vi "Main.vi"(11 "Error in":errorcluster) -> (15 "Error out":errorcluster)   [LabVIEW 2020, in "PSRR Monitor.lvlib"]
uses:
  PSRR Monitor.lvlib
  Typedefs/Queue operations.ctl
  Typedefs/Data Cluster.ctl
  Typedefs/Variant cluster.ctl
  Typedefs/User LV2 operations.ctl
  Typedefs/User LV2 data.ctl
  <vilib>/Utility/config.llb/Read Key (I32).vi
  <vilib>/Utility/config.llb/Read Key (Boolean).vi
  SubVI/Error log.vi
  <vilib>/Utility/config.llb/Write Key (I32).vi
  <vilib>/Utility/config.llb/Write Key (Boolean).vi
  <vilib>/Utility/config.llb/NI_LVConfig.lvlib
panel:
  out "Obtained PSRR":i32(graph)
  in  "Error Log":bool
  in  "Exit":bool
  out "Description":string
  out "Time":string
  out "Type":string
  out "Error Code":i32
  out "Last Read PSRR (dB)":i32
  in  "Wait Time(sec)":i32 min=2 step=1
  out "Error?":bool
  # "PSRR MONITOR"
  # "Power Supply Rejection Ratio"
  # "Last Error Details"
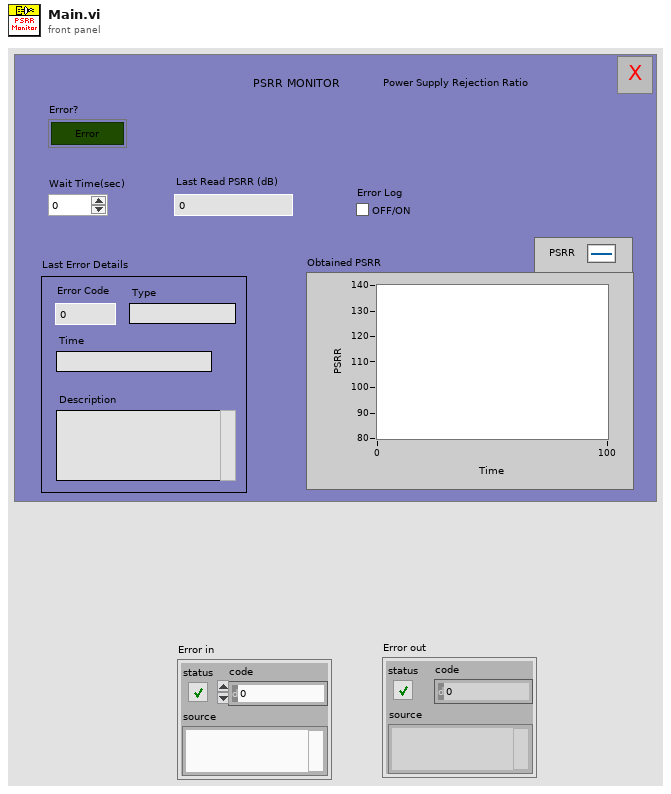
[diagram p1: front panel]
types:
  T1 = typedef "PSRR Monitor.lvlib/User LV2 operations.ctl" = enum16{"Destroy", "Get ref", "Generate", "Create"}
  T2 = typedef "PSRR Monitor.lvlib/Variant cluster.ctl" = cluster{"State":string, "Data":variant}
  T3 = typedef "PSRR Monitor.lvlib/Queue operations.ctl" = enum16{"Create", "Enqueue", "Enstack", "Dequeue", "Flush", "Release "}
  T4 = typedef "PSRR Monitor.lvlib/Data Cluster.ctl" = cluster{"Error?":bool, "Exit":bool, "Error log":bool, "Type":string, "Time":string, "Description":string, "Wait Time":i32, "Last Read PSRR":i32, "Error code":i32, "Obtained PSRR":i32, "Start/Stop Timer":bool, "Start time":dbl, "Path":path, "Passive count":dbl, "Other error count":dbl}
  T5 = typedef "PSRR Monitor.lvlib/User LV2 data.ctl" = cluster{"Exit":bool}
  T6 = typedef "NI_LVConfig.lvlib/Config Data RefNum.ctl" = refnum<k1>
  T7 = enum32{"Bad", "Idle", "Run top level", "Running"}
  T8 = typedef "PSRR Monitor.lvlib/Error Details.ctl" = cluster{"Error Code":i32, "Error Type":string, "Time":string, "Description":string, "PSRR":i32}
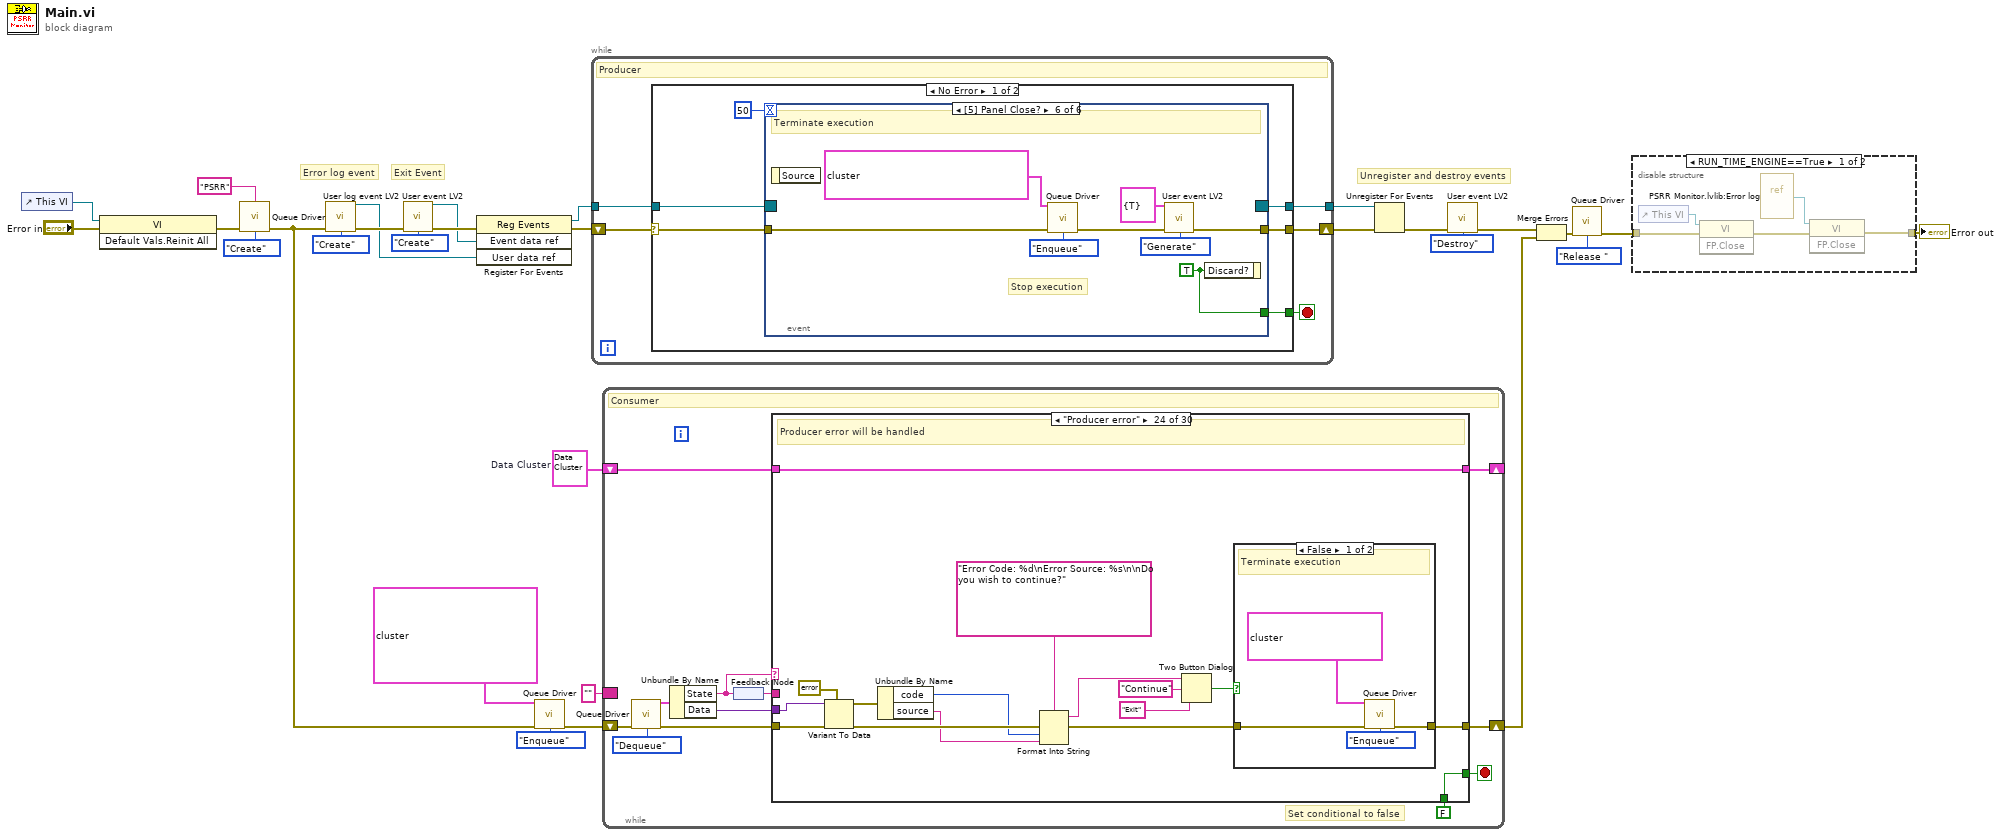
[diagram p0: block diagram]
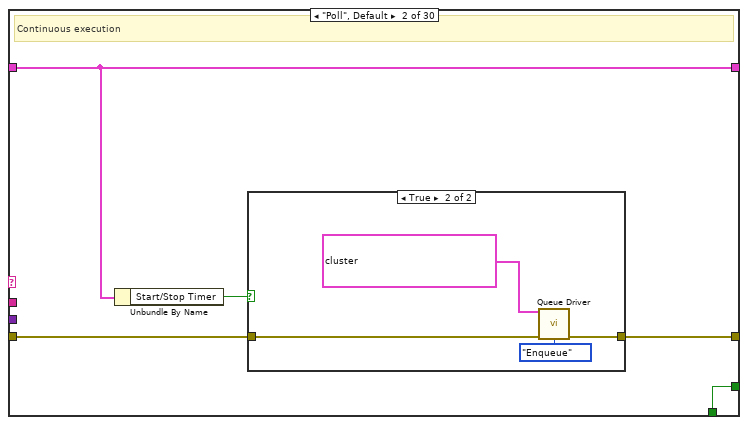
[diagram p4: hidden frame]
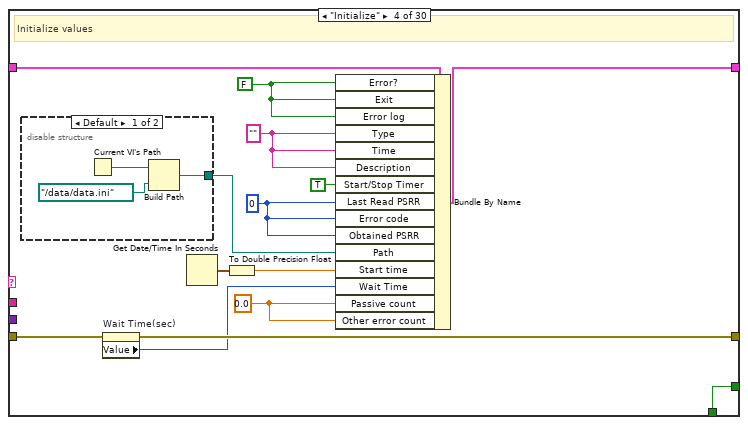
[diagram p7: hidden frame]
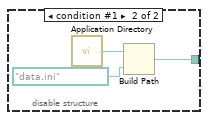
[diagram p8: hidden frame]
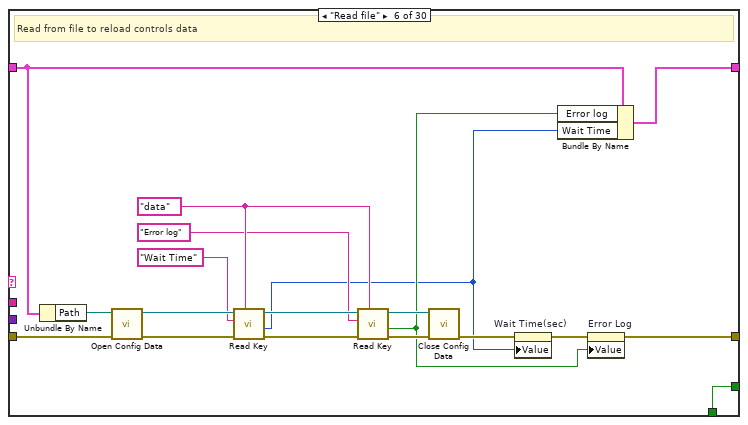
[diagram p10: hidden frame]
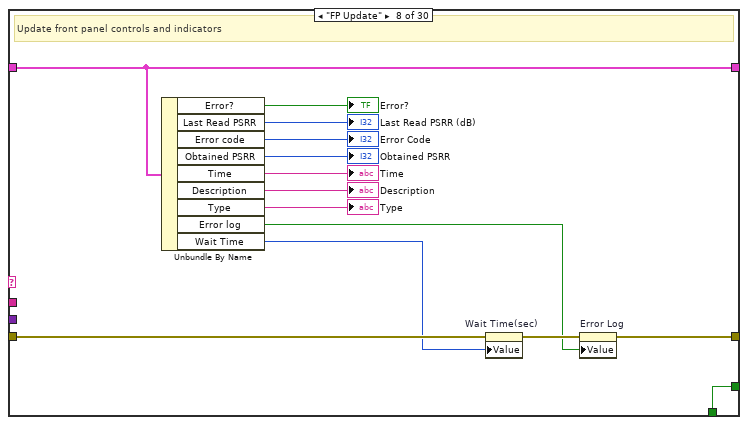
[diagram p12: hidden frame]
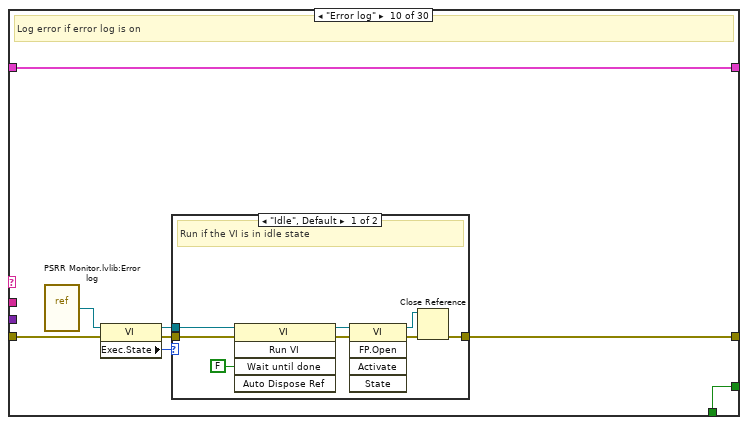
[diagram p14: hidden frame]
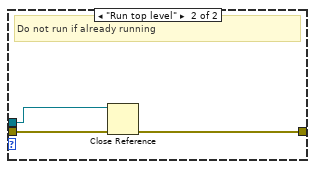
[diagram p15: hidden frame]
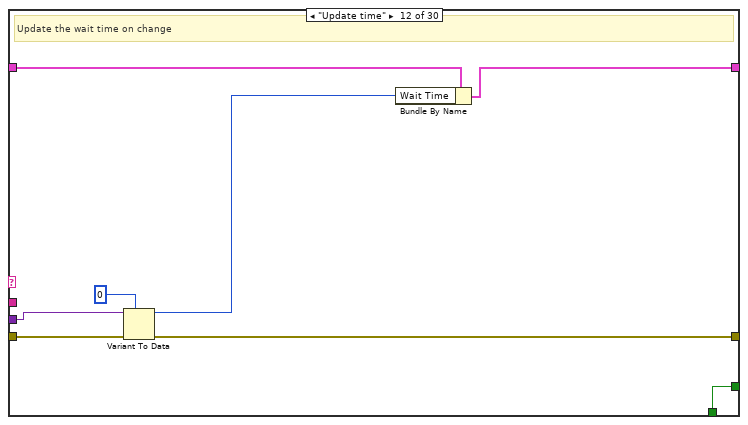
[diagram p17: hidden frame]
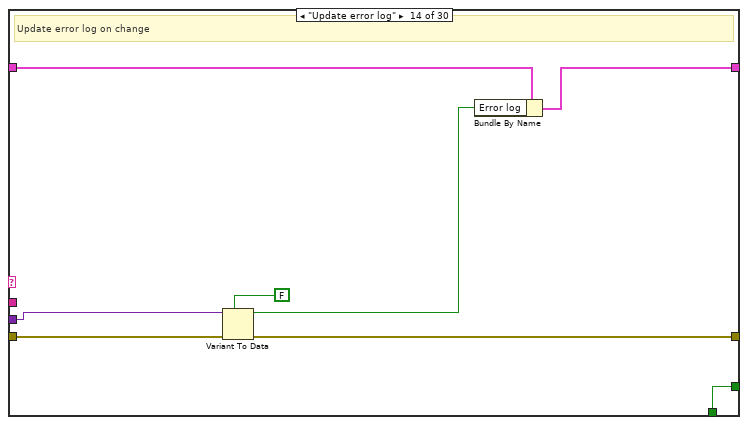
[diagram p19: hidden frame]
diagram:
  w24 = T4 {"Error?"=FALSE, "Exit"=FALSE, "Error log"=FALSE, "Type"="", "Time"="", "Description"="", "Wait Time"=0, "Last Read PSRR"=0, "Error code"=0, "Obtained PSRR"=0, "Start/Stop Timer"=FALSE, "Start time"=0.0, "Path"=path "", "Passive count"=0.0, "Other error count"=0.0}  # Data Cluster
  # "Unregister and destroy events"
  # "Exit Event"
  # "Error log event"
  n1 = control-ref of="This VI"() -> (w17:refnum<vi>)
  n2 = invoke class="VI" method="Default Vals.Reinit All"(reference=w17, error in="Error in") -> (error out=w15:errorcluster)  [unwired: 1 in, 2 out]
  n3 = call "Queue Driver.vi"("Name"="PSRR", "Error in"=w15, "Queue Operations"=Queue_operations."Create") -> ("Error out"=w3:errorcluster)  [unwired: 11 in, 1 out]
  n4 = call "User log event LV2.vi"("Error in"=w3, "Operation"=User_LV2_operations."Create") -> ("User data ref"=w1:refnum<user-event>, "Error out"=w2:errorcluster)  [unwired: 12 in]
  n5 = call "User event LV2.vi"("Error in"=w2, "Operation"=User_LV2_operations."Create") -> ("Event data ref"=w11:refnum<user-event>, "Error out"=w13:errorcluster)  [unwired: 12 in]
  n6 = register-events(error in=w13, w11, w1) -> (reference out=w10:refnum<event-registration>, error out=w12:errorcluster)  [unwired: 1 in]
  n7 = call "Queue Driver.vi"("State and data"=T2[] [{"State"="Initialize", "Data"=variant}, {"State"="Read file", "Data"=variant}, {"State"="FP Update", "Data"=variant}, {"State"="Error log", "Data"=variant}], "Error in"=w3, "Queue Operations"=Queue_operations."Enqueue") -> ("Error out"=w26:errorcluster)  [unwired: 11 in, 1 out]
  n8 = while {
    shift-right: [w33] -> w9
    shift-left: w12 -> [w34]
    tunnel: w10 -> [w31]
    tunnel: [w30] -> w8
    stop <- w32 stop-if-true
    # "Producer"
    n9 = case shown="No Error" w34 {
      selector: w34 -> [w38 w81]
      tunnel: [w39 w87] -> w33
      tunnel: [w37 FALSE ("Discard?")] -> w32
      tunnel: w31 -> [w36 w79]
      tunnel: [w35 w79] -> w30
      frame No Error {
        n10 = event shown="[5] Panel Close?" {
          selector: w36 -> [w41 _ _ _ _ _]
          dyn-events: [w41 _ _ _ _ _] -> w35
          timeout: 50 -> [_ _ _ _ _ _]
          tunnel: [w43 w50 w55 w65 w66 w71] -> w39
          tunnel: w38 -> [w43 w51 w56 w65 w68 w76]
          tunnel: [FALSE ("Discard?") FALSE ("Discard?") FALSE ("Discard?") w64 TRUE ("Discard?") w78] -> w37
          event Timeout {
            n11 = event-data() -> ()  [unwired: 1 in, 1 out]
          }
          event "Wait Time(sec)": Value Change {
            # "Enqueue state on value change"
            n12 = event-data() -> ("NewVal"=w49:i32)  [unwired: 1 in]
            n13 = To Variant(anything=w49) -> (Variant=w47:variant)
            n14 = Bundle By Name(cluster=T2 {"State"="", "Data"=variant} ("Dequeued output"), "State"="Update time", "Data"=w47) -> (w45:T2)
            n15 = Build Array(w45) -> (w44:T2[])
            n16 = call "Queue Driver.vi"("State and data"=w44, "Error in"=w51, "Queue Operations"=Queue_operations."Enqueue") -> ("Error out"=w50:errorcluster)  [unwired: 11 in, 1 out]
          }
          event "Error Log": Value Change {
            # "Update error log state on change"
            n17 = event-data() -> ("NewVal"=w59:bool)  [unwired: 1 in]
            n18 = To Variant(anything=w59) -> (Variant=w61:variant)
            n19 = Bundle By Name(cluster=T2 {"State"="", "Data"=variant} ("Dequeued output"), "State"="Update error log", "Data"=w61) -> (w58:T2)
            n20 = Build Array(w58) -> (w54:T2[])
            n21 = call "Queue Driver.vi"("State and data"=w54, "Error in"=w56, "Queue Operations"=Queue_operations."Enqueue") -> ("Error out"=w55:errorcluster)  [unwired: 11 in, 1 out]
          }
          event User Event {
            # "Event for critical error"
            n22 = event-data() -> ("Exit"=w64:bool)  [unwired: 1 in]
          }
          event "Exit": Value Change {
            # "Stop execution"
            # "Terminate execution"
            n23 = event-data() -> ()  [unwired: 1 in, 1 out]
            n24 = call "Queue Driver.vi"("State and data"=T2[] [{"State"="Write file", "Data"=variant}, {"State"="Exit", "Data"=variant}], "Error in"=w68, "Queue Operations"=Queue_operations."Enqueue") -> ("Error out"=w66:errorcluster)  [unwired: 11 in, 1 out]
          }
          event Panel Close? {
            w78 = TRUE ("Discard?")
            # "Stop execution"
            # "Terminate execution"
            n25 = event-data() -> ()  [unwired: 1 in, 1 out]
            n26 = call "Queue Driver.vi"("State and data"=T2[] [{"State"="Write file", "Data"=variant}, {"State"="Exit", "Data"=variant}], "Error in"=w76, "Queue Operations"=Queue_operations."Enqueue") -> ("Error out"=w72:errorcluster)  [unwired: 11 in, 1 out]
            n27 = call "User event LV2.vi"("Event data"=T5 {"Exit"=TRUE}, "Error in"=w72, "Operation"=User_LV2_operations."Generate") -> ("Error out"=w71:errorcluster)  [unwired: 11 in, 1 out]
            n28 = event-data("Discard?"=w78) -> ()  [unwired: 1 in, 1 out]
          }
        }
      }
      frame Error {
        n29 = To Variant(anything=w81) -> (Variant=w80:variant)
        n30 = Bundle By Name(cluster=T2 {"State"="", "Data"=variant} ("Dequeued output"), "State"="Producer error", "Data"=w80) -> (w84:T2)
        n31 = call <vilib>:"Clear Errors.vi"("error in (no error)"=w81) -> ("error out"=w86:errorcluster)  [unwired: 5 in, 1 out]
        n32 = Build Array(w84) -> (w83:T2[])
        n33 = call "Queue Driver.vi"("State and data"=w83, "Error in"=w86, "Queue Operations"=Queue_operations."Enqueue") -> ("Error out"=w87:errorcluster)  [unwired: 11 in, 1 out]
      }
    }
  }
  n34 = while {
    shift-right: [w93] -> w23
    shift-left: w26 -> [w100]
    border: "" ("State") -> [_]
    shift-right: [w94] -> _
    shift-left: w24 -> [w95]
    stop <- w92 stop-if-true
    # "Set conditional to false"
    # "Consumer"
    n35 = call "Queue Driver.vi"("Error in"=w100, "Queue Operations"=Queue_operations."Dequeue") -> ("Dequeued output"=w99:T2, "Error out"=w97:errorcluster)  [unwired: 12 in]
    n36 = Unbundle By Name(w99) -> ("State"=w90:string, "Data"=w98:variant)
    n37 = feedback-in #1(w90) -> ()
    n38 = feedback #1() -> (w96:string)
    n39 = case shown="\"Producer error\"" w90 {
      tunnel: w98 -> [_ _ _ _ _ _ _ _ _ _ _ w203 _ w216 _ _ _ _ _ _ _ _ _ w410 _ _ _ _ _ _]
      tunnel: w97 -> [w103 w108 w116 w120 w139 w158 w161 w167 w178 w184 w200 w206 w211 w218 w222 w230 w243 w267 w278 w339 w362 w383 w397 w411 w421 w427 w443 w460 w463 w466]
      tunnel: w95 -> [w104 w106 w117 w131 w140 w144 w162 w175 w179 w187 w201 w208 w212 w215 w223 w225 w234 w268 w281 w332 w360 w390 w398 w414 w422 w436 w444 w457 w464 w472]
      tunnel: [w104 w106 w117 w127 w140 w143 w162 w175 w179 w187 w201 w207 w212 w214 w223 w224 w240 w268 w280 w331 w358 w390 w398 w414 w422 w436 w444 w457 w464 w472] -> w94
      tunnel: [w103 w107 w116 w119 w139 w145 w161 w165 w178 w180 w200 w205 w211 w217 w222 w230 w242 w267 w282 w338 w361 w384 w397 w399 w421 w424 w443 w458 w463 w469] -> w93
      tunnel: [w102 w109 w115 w126 w138 w159 w160 w176 w177 w186 w199 w209 w210 w220 w221 w229 w231 w266 w284 w340 w365 w389 w396 w413 w420 w435 w442 w461 w462 TRUE] -> w92
      tunnel: FALSE -> [w102 w109 w115 w126 w138 w159 w160 w176 w177 w186 w199 w209 w210 w220 w221 w229 w231 w266 w284 w340 w365 w389 w396 w413 w420 w435 w442 w461 w462 _]
      tunnel: w96 -> [_ _ _ _ _ _ _ _ _ _ _ _ _ _ _ _ _ _ _ _ _ _ _ _ _ w428 _ _ _ _]
      frame "/***Application related***/" {
      }
      frame "Poll", Default {
        # "Continuous execution"
        n40 = Unbundle By Name(w106) -> ("Start/Stop Timer"=w105:bool)
        n41 = case shown="True" w105 {
          tunnel: w108 -> [w110 w113]
          tunnel: [w110 w112] -> w107
          frame False {
          }
          frame True {
            n42 = call "Queue Driver.vi"("State and data"=T2[] [{"State"="Get Elapsed Time", "Data"=variant}, {"State"="FP Update", "Data"=variant}], "Error in"=w113, "Queue Operations"=Queue_operations."Enqueue") -> ("Error out"=w112:errorcluster)  [unwired: 11 in, 1 out]
          }
        }
      }
      frame "/***Initialize***/" {
      }
      frame "Initialize" {
        w122 = 0.0 ("Passive count")
        w128 = "" ("Type")
        w129 = FALSE ("Error?")
        w130 = 0 ("Last Read PSRR")
        # "Initialize values"
        n43 = disable-structure shown="Default" {
          disable-tunnel: [w132 w136] -> w123
          frame condition #0 (active) {
            n44 = Current VI's Path() -> (path=w134:path)
            n45 = Build Path(base path=w134, name or relative path=path "../data/data.ini") -> (appended path=w132:path)
          }
          frame condition #1 {
            n46 = call <vilib>:"Application Directory.vi"() -> ("Application Directory"=w135:path)
            n47 = Build Path(base path=w135, name or relative path=path "data.ini") -> (appended path=w136:path)
          }
        }
        n48 = property on="Wait Time(sec)" class="DigNum (strict)"(error in=w120) -> (error out=w119:errorcluster, "Value"=w118:i32)  [unwired: 1 in, 1 out]
        n49 = Get Date/Time In Seconds() -> (seconds since 1Jan1904=w125:timestamp)
        n50 = To Double Precision Float(number=w125) -> (double precision float=w124:dbl)
        n51 = Bundle By Name(cluster=w131, "Error?"=w129, "Exit"=w129, "Error log"=w129, "Type"=w128, "Time"=w128, "Description"=w128, "Start/Stop Timer"=TRUE, "Last Read PSRR"=w130, "Error code"=w130, "Obtained PSRR"=w130, "Path"=w123, "Start time"=w124, "Wait Time"=w118, "Passive count"=w122, "Other error count"=w122) -> (w127:T4)
      }
      frame "/***Read from file ***/" {
      }
      frame "Read file" {
        w150 = "data" ("section")
        # "Read from file to reload controls data"
        n52 = Unbundle By Name(w144) -> ("Path"=w151:path)
        n53 = call <vilib>:"Open Config Data.vi"("error in (no error)"=w158, "configuration file path"=w151) -> ("error out"=w157:errorcluster, "refnum"=w154:T6)  [unwired: 7 in, 1 out]
        n54 = call-poly <vilib>:"Read Key.vi"("section"=w150, "error in (no error)"=w157, "key"="Wait Time", "refnum"=w154) -> ("error out"=w156:errorcluster, "value"=w141:i32, "refnum out"=w153:T6)  [unwired: 4 in, 1 out]
        n55 = call-poly <vilib>:"Read Key.vi"("section"=w150, "error in (no error)"=w156, "key"="Error log", "refnum"=w153) -> ("error out"=w155:errorcluster, "value"=w142:bool, "refnum out"=w152:T6)  [unwired: 4 in, 1 out]
        n56 = call <vilib>:"Close Config Data.vi"("error in (no error)"=w155, "refnum"=w152) -> ("error out"=w147:errorcluster)  [unwired: 8 in, 1 out]
        n57 = property on="Wait Time(sec)" class="DigNum (strict)"(error in=w147, "Value"=w141) -> (error out=w146:errorcluster)  [unwired: 1 in, 1 out]
        n58 = Bundle By Name(cluster=w144, "Error log"=w142, "Wait Time"=w141) -> (w143:T4)
        n59 = property on="Error Log" class="Bool (strict)"(error in=w146, "Value"=w142) -> (error out=w145:errorcluster)  [unwired: 1 in, 1 out]
      }
      frame "/***FP Related***/" {
      }
      frame "FP Update" {
        # "Update front panel controls and indicators"
        n60 = Unbundle By Name(w175) -> ("Error?"=→"Error?":bool, "Last Read PSRR"=→"Last Read PSRR (dB)":i32, "Error code"=→"Error Code":i32, "Obtained PSRR"=→"Obtained PSRR":i32, "Time"=→"Time":string, "Description"=→"Description":string, "Type"=→"Type":string, "Error log"=w163:bool, "Wait Time"=w164:i32)
        n61 = property on="Wait Time(sec)" class="DigNum (strict)"(error in=w167, "Value"=w164) -> (error out=w166:errorcluster)  [unwired: 1 in, 1 out]
        n62 = property on="Error Log" class="Bool (strict)"(error in=w166, "Value"=w163) -> (error out=w165:errorcluster)  [unwired: 1 in, 1 out]
      }
      frame "/***Error log***/" {
      }
      frame "Error log" {
        # "Log error if error log is on"
        n63 = vi-ref "PSRR Monitor.lvlib:Error log.vi"() -> (w185:refnum<vi>)
        n64 = property class="VI"(reference=w185, error in=w184) -> (reference out=w181:refnum<vi>, error out=w182:errorcluster, "Exec.State"=w183:T7)
        n65 = case shown="\"Idle\", Default" w183 {
          tunnel: w182 -> [w195 w197]
          tunnel: w181 -> [w193 w198]
          tunnel: [w192 w196] -> w180
          frame "Idle", Default {
            # "Run if the VI is in idle state"
            n66 = invoke class="VI" method="Run VI"(reference=w193, error in=w195, "Wait until done"=FALSE ("Wait Until Done")) -> (reference out=w189:refnum<vi>, error out=w191:errorcluster)  [unwired: 2 in, 3 out]
            n67 = invoke class="VI" method="FP.Open"(reference=w189, error in=w191) -> (reference out=w188:refnum<vi>, error out=w190:errorcluster)  [unwired: 3 in, 3 out]
            n68 = Close Reference(reference=w188, error in (no error)=w190) -> (error out=w192:errorcluster)
          }
          frame "Run top level" {
            # "Do not run if already running"
            n69 = Close Reference(reference=w198, error in (no error)=w197) -> (error out=w196:errorcluster)
          }
        }
      }
      frame "/*** Update wait time***/" {
      }
      frame "Update time" {
        # "Update the wait time on change"
        n70 = Variant To Data(error in=w206, type=0 ("NewVal"), Variant=w203) -> (data=w204:i32, error out=w205:errorcluster)
        n71 = Bundle By Name(cluster=w208, "Wait Time"=w204) -> (w207:T4)
      }
      frame "/***Update error log***/" {
      }
      frame "Update error log" {
        # "Update error log on change"
        n72 = Variant To Data(error in=w218, type=FALSE, Variant=w216) -> (data=w213:bool, error out=w217:errorcluster)
        n73 = Bundle By Name(cluster=w215, "Error log"=w213) -> (w214:T4)
      }
      frame "/***Timer Related***/" {
      }
      frame "Start Timer" {
        # "Start timer operation"
        n74 = Get Date/Time In Seconds() -> (seconds since 1Jan1904=w227:timestamp)
        n75 = To Double Precision Float(number=w227) -> (double precision float=w228:dbl)
        n76 = Bundle By Name(cluster=w225, "Start/Stop Timer"=TRUE, "Start time"=w228) -> (w224:T4)
      }
      frame "Get Elapsed Time" {
        # "Get elapsed time and call error classifier based on time"
        n77 = Unbundle By Name(w234) -> ("Start time"=w246:dbl, "Wait Time"=w244:i32)
        n78 = Get Date/Time In Seconds() -> (seconds since 1Jan1904=w247:timestamp)
        n79 = To Double Precision Float(number=w247) -> (double precision float=w245:dbl)
        n80 = Subtract(x=w245, y=w246) -> (x-y=w232:dbl)
        n81 = To Double Precision Float(number=w244) -> (double precision float=w233:dbl)
        n82 = Greater?(x=w232, y=w233) -> (0:w241:bool)
        n83 = case shown="True" w241 {
          tunnel: w243 -> [w254 w257]
          tunnel: [w254 w265] -> w242
          tunnel: [w252 w263] -> w239
          tunnel: [w251 w262] -> w238
          tunnel: [w250 w261] -> w237
          tunnel: [w249 w260] -> w236
          tunnel: [w248 w259] -> w235
          tunnel: w234 -> [w253 _]
          frame False {
            n84 = Unbundle By Name(w253) -> ("Error code"=w252:i32, "Type"=w251:string, "Time"=w250:string, "Description"=w249:string, "Obtained PSRR"=w248:i32)
          }
          frame True {
            n85 = call "Queue Driver.vi"("State and data"=T2[] [{"State"="FP Update", "Data"=variant}, {"State"="Error classifier", "Data"=variant}, {"State"="Start Timer", "Data"=variant}], "Error in"=w257, "Queue Operations"=Queue_operations."Enqueue") -> ("Error out"=w256:errorcluster)  [unwired: 11 in, 1 out]
            n86 = call "Error classifier.vi"("Error in"=w256) -> ("Classified Ouput Error"=w264:T8, "Error out"=w265:errorcluster)  [unwired: 13 in]
            n87 = Unbundle By Name(w264) -> ("Error Code"=w263:i32, "Error Type"=w262:string, "Time"=w261:string, "Description"=w260:string, "PSRR"=w259:i32)
          }
        }
        n88 = Bundle By Name(cluster=w234, "Error code"=w239, "Type"=w238, "Time"=w237, "Description"=w236, "Obtained PSRR"=w235) -> (w240:T4)
      }
      frame "/*** PSRR Error Related***/" {
      }
      frame "Error classifier" {
        # "Call error state based on error"
        n89 = Unbundle By Name(w281) -> ("Type"=w283:string, "Error log"=w269:bool, "Time"=w275:string, "Error code"=w272:i32, "Description"=w276:string, "Type"=w274:string)
        n90 = Number To Decimal String(number=w272) -> (decimal integer string=w277:string)  [unwired: 1 in]
        n91 = Not Equal To 0?(x=w272) -> (x != 0?=w270:bool)
        n92 = Build Array(w275, w277, w276, w274) -> (w273:string[])
        n93 = And(x=w269, y=w270) -> (x .and. y?=w271:bool)
        n94 = case shown="True" w271 {
          tunnel: [w285 w288] -> w279
          tunnel: w278 -> [w285 w289]
          tunnel: w273 -> [_ w287]
          frame False {
          }
          frame True {
            n95 = Build Array(w287) -> (w286:string[][])
            n96 = call "User log event LV2.vi"("User Data"=w286, "Error in"=w289, "Operation"=User_LV2_operations."Generate") -> ("Error out"=w288:errorcluster)  [unwired: 11 in, 1 out]
          }
        }
        n97 = case shown="\"Unknown Error\"" w283 {
          tunnel: w279 -> [w296 w299 w304 w313 w322]
          tunnel: [w295 w298 w310 w319 w328] -> w282
          tunnel: w281 -> [w293 w302 w308 w316 w326]
          tunnel: [w292 w301 w307 w317 w325] -> w280
          frame "", Default {
            # "No Error"
            n98 = Bundle By Name(cluster=w293, "Error?"=FALSE) -> (w292:T4)
            n99 = property on="Error?" class="Bool (strict)"(error in=w296, "BoolText.Text"="No Error" ("Boolean Text.Text")) -> (error out=w295:errorcluster)  [unwired: 1 in, 1 out]
          }
          frame "Warning" {
            # "Warning case"
            n100 = property on="Error?" class="Bool (strict)"(error in=w299, "BoolText.Text"="Warning" ("Boolean Text.Text")) -> (error out=w298:errorcluster)  [unwired: 1 in, 1 out]
            n101 = Bundle By Name(cluster=w302, "Error?"=TRUE) -> (w301:T4)
          }
          frame "Critical" {
            # "Critical Error"
            n102 = property on="Error?" class="Bool (strict)"(error in=w304, "BoolText.Text"="Error" ("Boolean Text.Text")) -> (error out=w303:errorcluster)  [unwired: 1 in, 1 out]
            n103 = Bundle By Name(cluster=w308, "Error?"=TRUE) -> (w307:T4)
            n104 = call "Queue Driver.vi"("State and data"=T2[] [{"State"="Critical", "Data"=variant}], "Error in"=w303, "Queue Operations"=Queue_operations."Enqueue") -> ("Error out"=w310:errorcluster)  [unwired: 11 in, 1 out]
          }
          frame "Passive" {
            # "Passive error"
            n105 = property on="Error?" class="Bool (strict)"(error in=w313, "BoolText.Text"="Error" ("Boolean Text.Text")) -> (error out=w312:errorcluster)  [unwired: 1 in, 1 out]
            n106 = Bundle By Name(cluster=w316, "Error?"=TRUE) -> (w317:T4)
            n107 = call "Queue Driver.vi"("State and data"=T2[] [{"State"="Passive", "Data"=variant}], "Error in"=w312, "Queue Operations"=Queue_operations."Enqueue") -> ("Error out"=w319:errorcluster)  [unwired: 11 in, 1 out]
          }
          frame "Unknown Error" {
            # "Unknown error"
            n108 = property on="Error?" class="Bool (strict)"(error in=w322, "BoolText.Text"="Error" ("Boolean Text.Text")) -> (error out=w321:errorcluster)  [unwired: 1 in, 1 out]
            n109 = Bundle By Name(cluster=w326, "Error?"=TRUE) -> (w325:T4)
            n110 = call "Queue Driver.vi"("State and data"=T2[] [{"State"="Unknown Error", "Data"=variant}], "Error in"=w321, "Queue Operations"=Queue_operations."Enqueue") -> ("Error out"=w328:errorcluster)  [unwired: 11 in, 1 out]
          }
        }
      }
      frame "Unknown Error" {
        # "Third occurrence of error"
        # "Unknown error information for user"
        n111 = Unbundle By Name(w332) -> ("Description"=w334:string, "Other error count"=w337:dbl, "Other error count"=w330:dbl)
        n112 = Greater Or Equal?(x=w337, y=3.0) -> (x >= y?=w335:bool)
        n113 = case shown="False" w335 {
          tunnel: w339 -> [w345 w357]
          tunnel: [w345 w357] -> w338
          tunnel: w334 -> [_ w356]
          tunnel: "Occurred with code at  " ("string") -> [_ w355]
          tunnel: w332 -> [w344 w351]
          tunnel: [w343 w350] -> w331
          tunnel: w330 -> [w341 _]
          frame False {
            # "Increment count"
            n114 = Increment(x=w341) -> (x+1=w342:dbl)
            n115 = Bundle By Name(cluster=w344, "Other error count"=w342) -> (w343:T4)
          }
          frame True {
            # "Count is 3 then create a pop up to user"
            n116 = Concatenate Strings(w355, w356) -> (w354:string)
            n117 = Two Button Dialog(message=w354, 1:"Acknowledge next" ("F button name (\"Cancel\")"), 2:"Continue" ("T button name (\"OK\")")) -> (T button?=w349:bool)
            n118 = Select(t=0.0, s=w349, f=3.0) -> (s? t:f=w346:dbl)
            n119 = Bundle By Name(cluster=w351, "Other error count"=w346) -> (w350:T4)
          }
        }
      }
      frame "Passive" {
        # "Passive information and acknowledgement from the user"
        n120 = Unbundle By Name(w360) -> ("Passive count"=w359:dbl)
        n121 = Greater Or Equal?(x=w359, y=3.0) -> (x >= y?=w363:bool)
        n122 = case shown="True" w363 {
          tunnel: w362 -> [w370 w380]
          tunnel: [w370 w380] -> w361
          tunnel: w360 -> [w369 w376]
          tunnel: w359 -> [w367 _]
          tunnel: [w366 w375] -> w358
          frame False {
            # "Continue"
            n123 = Increment(x=w367) -> (x+1=w368:dbl)
            n124 = Bundle By Name(cluster=w369, "Passive count"=w368) -> (w366:T4)
          }
          frame True {
            # "Pop up for user if error occurred thrice"
            n125 = Two Button Dialog(message="Passive error has occurred", 1:"Acknowledge next" ("F button name (\"Cancel\")"), 2:"Continue" ("T button name (\"OK\")")) -> (T button?=w373:bool)
            n126 = Select(t=0.0, s=w373, f=2.0) -> (s? t:f=w374:dbl)
            n127 = Bundle By Name(cluster=w376, "Passive count"=w374) -> (w375:T4)
          }
        }
      }
      frame "Critical" {
        # "Critical information for user"
        n128 = property on="Obtained PSRR" class="WFChart (strict)"(error in=w383, "History Data"=i32[] []) -> (error out=w382:errorcluster)  [unwired: 1 in, 1 out]
        n129 = Two Button Dialog(message="Critical Error has occurred", 1:"Exit" ("F button name (\"Cancel\")"), 2:"Continue" ("T button name (\"OK\")")) -> (T button?=w385:bool)
        n130 = case shown="True" w385 {
          tunnel: w382 -> [w391 w395]
          tunnel: [w393 w395] -> w384
          frame False {
            # "Exit if user press exit"
            n131 = call "Queue Driver.vi"("State and data"=T2[] [{"State"="Write file", "Data"=variant}, {"State"="Exit", "Data"=variant}], "Error in"=w391, "Queue Operations"=Queue_operations."Enqueue") -> ("Error out"=w393:errorcluster)  [unwired: 11 in, 1 out]
          }
          frame True {
            # "Continue"
          }
        }
      }
      frame "/***Producer error***/" {
      }
      frame "Producer error" {
        # "Producer error will be handled"
        n132 = Variant To Data(error in=w411, type=errorcluster {"status"=FALSE, "code"=0, "source"=""} ("Error out"), Variant=w410) -> (data=w408:errorcluster, error out=w407:errorcluster)
        n133 = Unbundle By Name(w408) -> ("code"=w406:i32, "source"=w405:string)
        n134 = Format Into String(format string="Error Code: %d\nError Source: %s\n\nDo you wish to continue?", error in=w407, w406, w405) -> (resulting string=w403:string, error out=w400:errorcluster)  [unwired: 1 in]
        n135 = Two Button Dialog(message=w403, 1:"Exit" ("F button name (\"Cancel\")"), 2:"Continue" ("T button name (\"OK\")")) -> (T button?=w404:bool)
        n136 = case shown="False" w404 {
          tunnel: w400 -> [w417 w419]
          tunnel: [w416 w419] -> w399
          frame False {
            # "Terminate execution"
            n137 = call "Queue Driver.vi"("State and data"=T2[] [{"State"="Write file", "Data"=variant}, {"State"="Exit", "Data"=variant}], "Error in"=w417, "Queue Operations"=Queue_operations."Enqueue") -> ("Error out"=w416:errorcluster)  [unwired: 11 in, 1 out]
          }
          frame True {
            # "Continue"
          }
        }
      }
      frame "/***Consumer Error***/" {
      }
      frame "Error" {
        # "Consumer error will be handled"
        n138 = Unbundle By Name(w427) -> ("code"=w432:i32, "source"=w426:string)
        n139 = call <vilib>:"Clear Errors.vi"("error in (no error)"=w427, "specific error code to clear (0: all)"=w432) -> ("error out"=w434:errorcluster)  [unwired: 4 in, 1 out]
        n140 = Format Into String(format string="Error occurred in state \"%s\"!!\nError Code: %d\nError Source: %s\n\nDo you wish to continue?", error in=w434, w428, w432, w426) -> (resulting string=w431:string, error out=w423:errorcluster)  [unwired: 1 in]
        n141 = Two Button Dialog(message=w431, 1:"Exit" ("F button name (\"Cancel\")"), 2:"Continue" ("T button name (\"OK\")")) -> (T button?=w425:bool)
        n142 = case shown="False" w425 {
          tunnel: [w437 w441] -> w424
          tunnel: w423 -> [w438 w441]
          frame False {
            # "Terminate execution"
            n143 = call "Queue Driver.vi"("State and data"=T2[] [{"State"="Write file", "Data"=variant}, {"State"="Exit", "Data"=variant}], "Error in"=w438, "Queue Operations"=Queue_operations."Enqueue") -> ("Error out"=w437:errorcluster)  [unwired: 11 in, 1 out]
          }
          frame True {
            # "Continue"
          }
        }
      }
      frame "/***Write file on exit***/" {
      }
      frame "Write file" {
        w452 = "data" ("section")
        # "Do not create a new file"
        # "Write back controls status to ini file"
        n144 = Unbundle By Name(w457) -> ("Error log"=w445:bool, "Wait Time"=w446:i32, "Path"=w456:path)
        n145 = call <vilib>:"Open Config Data.vi"("error in (no error)"=w460, "create file if necessary (T)"=FALSE, "configuration file path"=w456) -> ("error out"=w459:errorcluster, "refnum"=w455:T6)  [unwired: 6 in, 1 out]
        n146 = call-poly <vilib>:"Write Key.vi"("section"=w452, "error in (no error)"=w459, "value"=w446, "key"="Wait Time", "refnum"=w455) -> ("error out"=w454:errorcluster, "refnum out"=w451:T6)  [unwired: 4 in, 1 out]
        n147 = call-poly <vilib>:"Write Key.vi"("section"=w452, "error in (no error)"=w454, "value"=w445, "key"="Error log", "refnum"=w451) -> ("error out"=w453:errorcluster, "refnum out"=w450:T6)  [unwired: 4 in, 1 out]
        n148 = call <vilib>:"Close Config Data.vi"("error in (no error)"=w453, "refnum"=w450) -> ("error out"=w458:errorcluster)  [unwired: 8 in, 1 out]
      }
      frame "/***Exit***/" {
      }
      frame "Exit" {
        # "Stop execution"
        # "flush and terminate loop"
        n149 = call "User event LV2.vi"("Event data"=T5 {"Exit"=TRUE}, "Error in"=w466, "Operation"=User_LV2_operations."Generate") -> ("Error out"=w465:errorcluster)  [unwired: 11 in, 1 out]
        n150 = call "Queue Driver.vi"("Error in"=w465, "Queue Operations"=Queue_operations."Flush") -> ("Error out"=w469:errorcluster)  [unwired: 12 in, 1 out]
      }
    }
  }
  n151 = Unregister For Events(event registration refnum=w8, error in=w9) -> (error out=w6:errorcluster)
  n152 = call "User event LV2.vi"("Error in"=w6, "Operation"=User_LV2_operations."Destroy") -> ("Error out"=w5:errorcluster)  [unwired: 12 in, 1 out]
  n153 = Merge Errors(w5, w23) -> (w21:errorcluster)
  n154 = call "Queue Driver.vi"("Error in"=w21, "Queue Operations"=Queue_operations."Release ") -> ("Error out"=w20:errorcluster)  [unwired: 12 in, 1 out]
  n155 = disable-structure shown="RUN_TIME_ENGINE==True" {
    disable-tunnel: w20 -> [w477 w478]
    disable-tunnel: [w474 w478] -> w19
    frame condition #0 {
      n156 = control-ref of="This VI"() -> (w476:refnum<vi>)
      n157 = invoke class="VI" method="FP.Close"(reference=w476, error in=w477) -> (error out=w475:errorcluster)  [unwired: 1 in, 2 out]
      n158 = vi-ref "PSRR Monitor.lvlib:Error log.vi"() -> (w473:refnum<vi>)
      n159 = invoke class="VI" method="FP.Close"(reference=w473, error in=w475) -> (error out=w474:errorcluster)  [unwired: 1 in, 2 out]
    }
    frame condition #1 (active) {
    }
  }
  "Error out" <- w19
